vi "AODO-Set AO Gains.vi"(0 "Tasks":T1[](array[typedef]), 7 "Gains":dbl[](array[numeric]), 11 "error in (no error)":errorcluster) -> (4 "Tasks out":T1[](array[typedef]), 15 "error out":errorcluster)   [LabVIEW 2020]
uses:
  Typedefs/AODO-Task Specification.ctl
  <resource>/objmgr/daqmx.rc
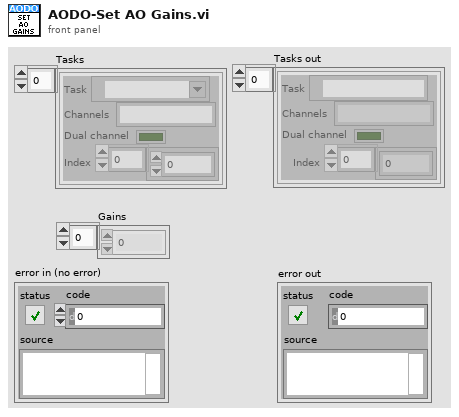
[diagram p1: front panel]
types:
  T1 = typedef "AODO-Task Specification.ctl" = cluster{"Task":refnum<k21>, "Channels":string, "Dual channel":bool, "Index":i32[]}
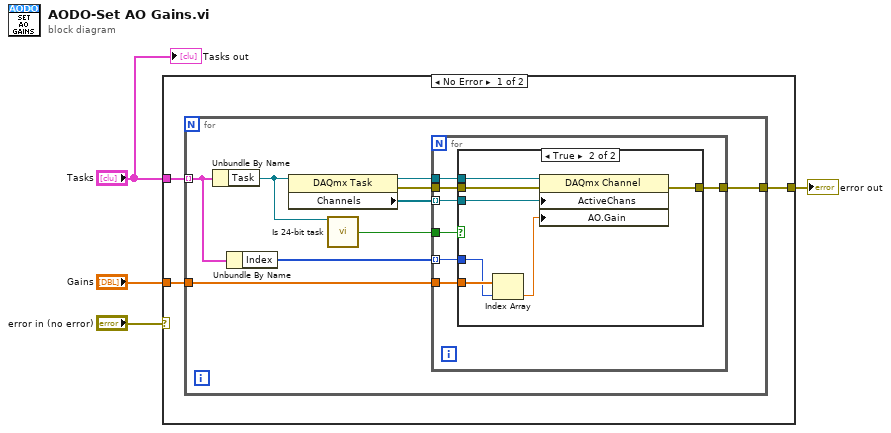
[diagram p0: block diagram]
diagram:
  n1 = case shown="No Error" "error in (no error)" {
    selector: "error in (no error)" -> [_ w31]
    tunnel: "Tasks" -> [w7 _]
    tunnel: "Gains" -> [w6 _]
    tunnel: [w5 w31] -> w2
    frame No Error {
      n2 = for {
        tunnel: w7 -> [w11] mode=indexing
        tunnel: w6 -> [w12]
        tunnel: [w9] -> w5
        n3 = Unbundle By Name(w11) -> ("Task"=w16:refnum<k21>)
        n4 = Unbundle By Name(w11) -> ("Index"=w10:i32[])
        n5 = property class="DAQmx Task"(reference=w16) -> (reference out=w15:refnum<k21>, error out=w8:errorcluster, "Channels"=w14:refnum<k21>[])  [unwired: 1 in]
        n6 = call "Is 24-bit task.vi"("task"=w16) -> ("is 24bit?"=w13:bool)  [unwired: 9 in, 5 out]
        n7 = for {
          tunnel: w15 -> [w23]
          tunnel: w14 -> [w22] mode=indexing
          tunnel: w13 -> [w21]
          tunnel: w12 -> [w20]
          tunnel: w10 -> [w19] mode=indexing
          tunnel: [w18] -> w9
          tunnel: w8 -> [w17]
          n8 = case shown="True" w21 {
            tunnel: w23 -> [_ w30]
            tunnel: w22 -> [_ w29]
            tunnel: w20 -> [_ w28]
            tunnel: w19 -> [_ w27]
            tunnel: [_ w25] -> w18
            tunnel: w17 -> [_ w24]
            frame False {
            }
            frame True {
              n9 = Index Array(array=w28, index=w27) -> (element=w26:dbl)
              n10 = property class="DAQmx Channel"(reference=w30, error in=w24, "ActiveChans"=w29, "AO.Gain"=w26) -> (error out=w25:errorcluster)  [unwired: 1 out]
            }
          }
        }
      }
    }
    frame Error {
    }
  }
  "error out" <- w2
  "Tasks out" <- "Tasks"
